vi "LabVIEW-CommEx_Bus_Interface_PWM_SPI_v1.1a_Scaled_6Apr2023.vi"() -> ()   [LabVIEW 2018]
uses:
  <vilib>/Instr/_visa.llb/VISA Set IO Buffer Mask.ctl
  <vilib>/Utility/error.llb/DialogType.ctl
  <vilib>/Instr/_visa.llb/VISA Configure Serial Port (Serial Instr).vi
panel:
  out "V_DC_In":dbl format="%.2f"
  out "V_Boost":dbl format="%.2f"
  out "V_Buck":dbl format="%.2f"
  out "V_Pot":dbl format="%.2f"
  in  "LED4_Intensity":dbl(slide)=100.0 scale=0.0..100.0
  in  "LED3_Intensity":dbl(slide)=50.0 scale=0.0..100.0
  in  "LED2_Intensity":dbl(slide)=25.0 scale=0.0..100.0
  in  "LED_BlinkPRD":dbl(slide)=75.0 scale=0.0..100.0
  in  "LED1_Intensity":dbl(slide)=12.5 scale=0.0..100.0
  in  "PWM_En":bool=TRUE
  out "error out 2":errorcluster={"status"=FALSE, "code"=1073676294, "source"="VISA Read in LabVIEW-Int_FPGA_CommExample_2Jun2019_v1.1a_2Jun2019.vi"}
  out "Reg_Array":u16[](array[numeric])=[1, 49151, 24576, 8192, 16384, 32768, 65535, 0, 0, 0, 0, 0, 0, 0, 0, 0, 0, 0, 0, 0, 0, 0, 0, 0, 0, 0, 0, 0, 0, 0, 0, 0, 0, 0, 0, 0, 0, 0, 0, 0, 0, 0, 0, 0, 0, 0, 0, 0, 0, 0, 0, 0, 0, 0, 0, 0, 0, 0, 0, 0, 0, 0, 0, 0] format="%x"
  out "Read_Packet":string
  out "CkSum":bool=TRUE
  out "Recieved Packet":string
  in  "flow control":u16(ring) items=["None"=0, "XON/XOFF"=1, "RTS/CTS"=2, "DTR/DSR"=4]
  in  "Input Buffer Size":u32=16484
  in  "stop 2":bool
  in  "timeout (ms)":u32=100000
  in  "stop bits":u16(ring)=10 items=["1.0"=10, "1.5"=15, "2.0"=20]
  in  "parity":u16(ring) items=["None", "Odd", "Even", "Mark", "Space"]
  in  "data bits":u16=8 min=5 max=8 step=1
  in  "VISA resource name":refnum<visa-resource-name>="COM4"
  in  "baud rate":u32=9600
  out "Cmd_Packet":string
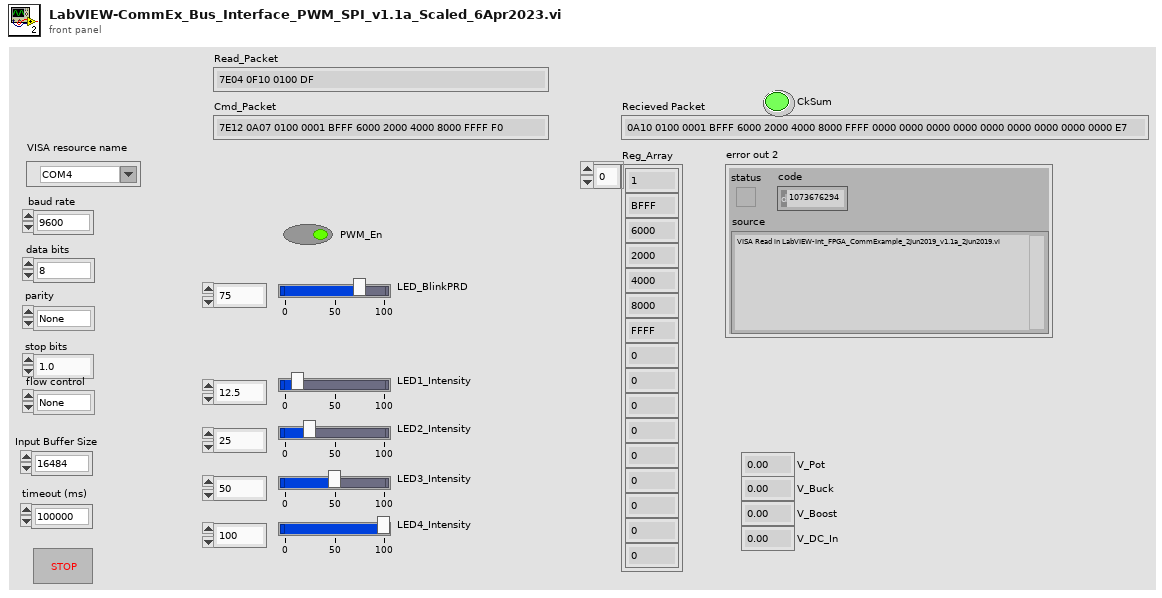
[diagram p1: front panel]
types:
  T1 = typedef "DialogType.ctl" = u16
  T2 = typedef "VISA Set IO Buffer Mask.ctl" = u16
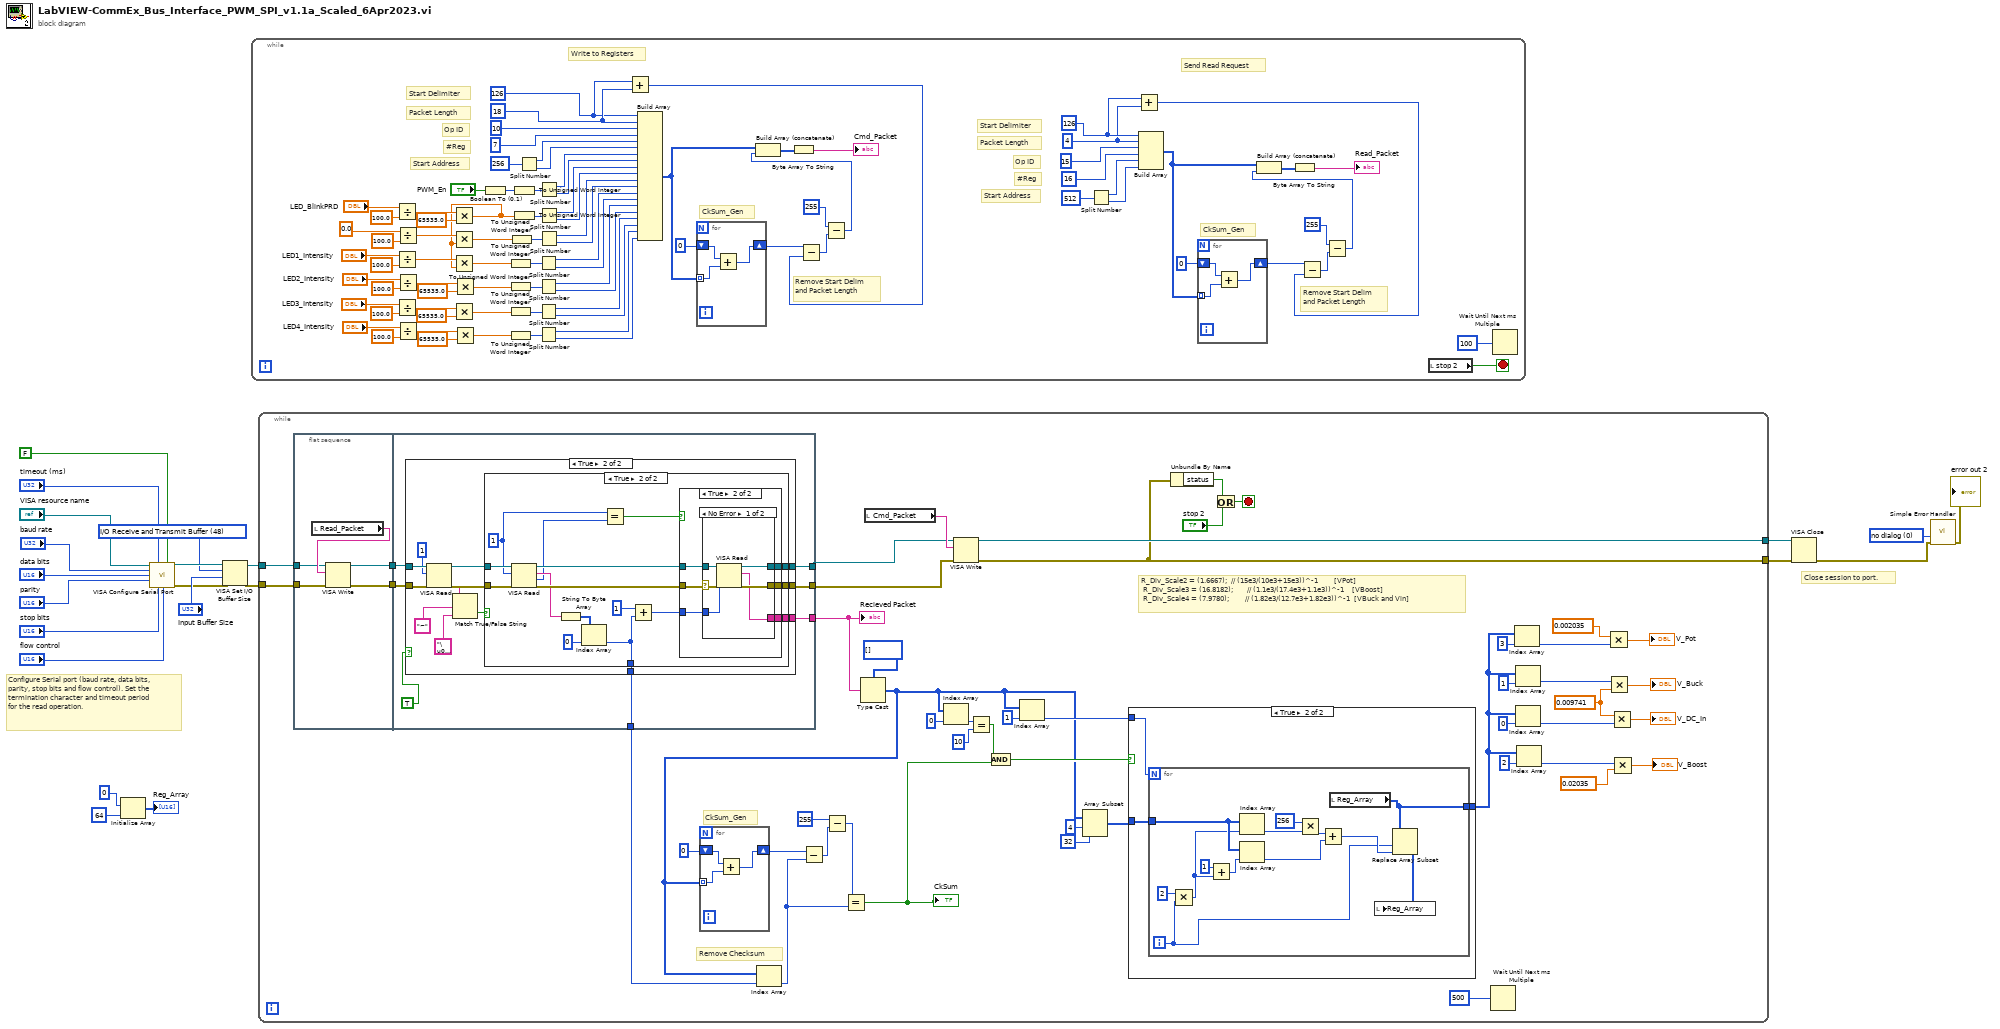
[diagram p0: block diagram]
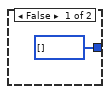
[diagram p2: hidden frame]
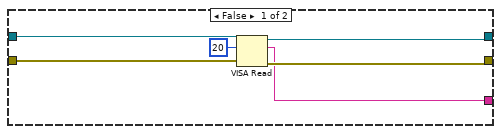
[diagram p3: hidden frame]
diagram:
  w2 = T1 0 items=["no dialog", "OK message", "continue or stop message", "OK message + warnings", "continue/stop + warnings"] ("type of dialog (OK msg:1)")
  w7 = T2 48 items=["I/O Receive Buffer"=16, "I/O Transmit Buffer"=32, "I/O Receive and Transmit Buffer"=48] ("Mask")
  # "Configure Serial port (baud rate, data bits, parity, stop bits and flow control). Set the termination character and timeout period for the read operation."
  # "Close session to port."
  n1 = Initialize Array(u16 0 ("element"), 64 ("dimension size")) -> (→"Reg_Array":u16[])
  n2 = call-poly "VISA Configure Serial Port"("VISA resource name"="VISA resource name", "timeout (10sec)"="timeout (ms)", "Enable Termination\nChar (T)"=FALSE, "baud rate (9600)"="baud rate", "data bits (8)"="data bits", "parity (0:none)"="parity", "stop bits (10: 1 bit)"="stop bits", "flow control (0:none)"="flow control") -> ("VISA resource name out"=w14:refnum<visa-resource-name>, "error out"=w13:errorcluster)  [unwired: 2 in, 4 out]
  n3 = VISA Set I/O Buffer Size(VISA resource name=w14, mask (16)=w7, size (4096)="Input Buffer Size", error in (no error)=w13) -> (VISA resource name out=w10:refnum<visa-resource-name>, error out=w11:errorcluster)
  n4 = while {
    stop <- w97 stop-if-true
    w26 = u8 4
    w27 = u8 126
    w80 = u8 18
    w79 = u8 126
    # "Write to Registers"
    # "Send Read Request"
    # "#Reg"
    # "Start Address"
    # "Start Delimiter"
    # "Packet Length"
    # "Op ID"
    # "Remove Start Delim\nand Packet Length"
    # "CkSum_Gen"
    # "Remove Start Delim\nand Packet Length"
    # "CkSum_Gen"
    # "#Reg"
    # "Start Address"
    # "Start Delimiter"
    # "Packet Length"
    # "Op ID"
    n5 = Divide(x="LED_BlinkPRD", y=100.0) -> (x/y=w60:dbl)
    n6 = Divide(x="LED1_Intensity", y=100.0) -> (x/y=w54:dbl)
    n7 = Divide(x="LED3_Intensity", y=100.0) -> (x/y=w43:dbl)
    n8 = Divide(x=0.0, y=100.0) -> (x/y=w57:dbl)
    n9 = Divide(x="LED2_Intensity", y=100.0) -> (x/y=w50:dbl)
    n10 = Divide(x="LED4_Intensity", y=100.0) -> (x/y=w38:dbl)
    n11 = Multiply(x=w60, y=65535.0 ("x")) -> (x*y=w23:dbl)
    n12 = Multiply(x=w57, y=w23) -> (x*y=w56:dbl)
    n13 = Multiply(x=w54, y=w23) -> (x*y=w53:dbl)
    n14 = Multiply(x=w43, y=65535.0 ("x")) -> (x*y=w41:dbl)
    n15 = Multiply(x=w50, y=65535.0 ("x")) -> (x*y=w47:dbl)
    n16 = Multiply(x=w38, y=65535.0 ("x")) -> (x*y=w35:dbl)
    n17 = Boolean To (0,1)(Boolean="PWM_En") -> (0, 1=w76:i16)
    n18 = To Unsigned Word Integer(number=w53) -> (unsigned 16bit integer=w93:u16)
    n19 = To Unsigned Word Integer(number=w47) -> (unsigned 16bit integer=w92:u16)
    n20 = To Unsigned Word Integer(number=w41) -> (unsigned 16bit integer=w46:u16)
    n21 = To Unsigned Word Integer(number=w35) -> (unsigned 16bit integer=w45:u16)
    n22 = To Unsigned Word Integer(number=w56) -> (unsigned 16bit integer=w94:u16)
    n23 = To Unsigned Word Integer(number=w76) -> (unsigned 16bit integer=w81:u16)
    n24 = To Unsigned Word Integer(number=w23) -> (unsigned 16bit integer=w107:u16)
    n25 = Split Number(x=u16 256) -> (hi(x)=w74:u8, lo(x)=w73:u8)
    n26 = Split Number(x=w93) -> (hi(x)=w66:u8, lo(x)=w65:u8)
    n27 = Split Number(x=w92) -> (hi(x)=w64:u8, lo(x)=w63:u8)
    n28 = Split Number(x=w46) -> (hi(x)=w34:u8, lo(x)=w33:u8)
    n29 = Split Number(x=w45) -> (hi(x)=w32:u8, lo(x)=w31:u8)
    n30 = Split Number(x=w81) -> (hi(x)=w72:u8, lo(x)=w71:u8)
    n31 = Split Number(x=w107) -> (hi(x)=w70:u8, lo(x)=w69:u8)
    n32 = Split Number(x=w94) -> (hi(x)=w68:u8, lo(x)=w67:u8)
    n33 = Add(x=w79, y=w80) -> (x+y=w78:u8)
    n34 = Build Array(w79, w80, u8 10, u8 7, w74, w73, w72, w71, w70, w69, w68, w67, w66, w65, w64, w63, w34, w33, w32, w31) -> (w104:u8[])
    n35 = for {
      tunnel: w104 -> [w111] mode=indexing
      shift-right: [w113] -> w96
      shift-left: u8 0 -> [w112]
      n36 = Add(x=w112, y=w111) -> (x+y=w113:u8)
    }
    n37 = Subtract(x=w96, y=w78) -> (x-y=w95:u8)
    n38 = Subtract(x=u8 255, y=w95) -> (x-y=w98:u8)
    n39 = Build Array (concatenate)(w104, w98) -> (w103:u8[])
    n40 = Byte Array To String(unsigned byte array=w103) -> (string=→"Cmd_Packet":string)
    n41 = Split Number(x=u16 512) -> (hi(x)=w29:u8, lo(x)=w28:u8)
    n42 = Add(x=w27, y=w26) -> (x+y=w25:u8)
    n43 = Build Array(w27, w26, u8 15, u8 16, w29, w28) -> (w90:u8[])
    n44 = for {
      tunnel: w90 -> [w108] mode=indexing
      shift-right: [w110] -> w85
      shift-left: u8 0 -> [w109]
      n45 = Add(x=w109, y=w108) -> (x+y=w110:u8)
    }
    n46 = Subtract(x=w85, y=w25) -> (x-y=w84:u8)
    n47 = Subtract(x=u8 255, y=w84) -> (x-y=w86:u8)
    n48 = Build Array (concatenate)(w90, w86) -> (w89:u8[])
    n49 = Byte Array To String(unsigned byte array=w89) -> (string=→"Read_Packet":string)
    n50 = local read "stop 2"() -> (w97:bool)
    n51 = Wait Until Next ms Multiple(millisecond multiple=u8 100) -> ()  [unwired: 1 out]
  }
  n52 = while {
    tunnel: w11 -> [w147]
    tunnel: w10 -> [w148]
    tunnel: [w152] -> w8
    tunnel: [w135] -> w9
    stop <- w162 stop-if-true
    w121 = 0.009741
    # "R_Div_Scale2 = (1.6667);\t\t// (15e3/(10e3+15e3))^-1        [VPot]\n\tR_Div_Scale3 = (16.8182);       // (1.1e3/(17.4e3+1.1e3))^-1    [VBoost]\n\tR_Div_Scale4 = (7.9780);        // (1.82e3/(12.7e3+1.82e3))^-1  [VBuck and Vin]"
    # "Remove Checksum"
    # "CkSum_Gen"
    n53 = flat-sequence {
      tunnel: [w184] -> w150
      tunnel: [w183] -> w149
      tunnel: w148 -> [w182]
      tunnel: w147 -> [w181]
      tunnel: [w192] -> w151
      tunnel: w150 -> [w191]
      tunnel: w149 -> [w190]
      tunnel: [w189] -> w146
      tunnel: [w188] -> w145
      tunnel: [w186] -> w138
      frame #0 {
        n54 = local read "Read_Packet"() -> (w185:string)
        n55 = VISA Write(VISA resource name=w182, write buffer=w185, error in (no error)=w181) -> (VISA resource name out=w184:refnum<visa-resource-name>, error out=w183:errorcluster)  [unwired: 1 out]
      }
      frame #1 {
        n56 = case shown="True" TRUE {
          tunnel: w190 -> [w197 w208]
          tunnel: w191 -> [w198 w206]
          tunnel: [w195 w211] -> w188
          tunnel: [w196 w210] -> w189
          tunnel: [w193 w209] -> w192
          tunnel: [_ w199] -> w186
          frame False {
            n57 = VISA Read(VISA resource name=w198, byte count=u32 20, error in (no error)=w197) -> (VISA resource name out=w196:refnum<visa-resource-name>, read buffer=w193:string, error out=w195:errorcluster)  [unwired: 1 out]
          }
          frame True {
            n58 = VISA Read(VISA resource name=w206, byte count=u32 1 ("millisecond multiple"), error in (no error)=w208) -> (VISA resource name out=w205:refnum<visa-resource-name>, read buffer=w203:string, error out=w207:errorcluster)  [unwired: 1 out]
            n59 = Match True/False String(2:"\u0000", 3:"~", 4:w203) -> (0:w201:bool)  [unwired: 1 out]
            n60 = case shown="True" w201 {
              tunnel: [w212 w229] -> w211
              tunnel: [w213 w228] -> w210
              tunnel: [_ w227] -> w209
              tunnel: w207 -> [w212 w226]
              tunnel: w205 -> [w213 w225]
              tunnel: [_ w214] -> w199
              frame False {
              }
              frame True {
                w218 = u32 1 ("byte count")
                n61 = VISA Read(VISA resource name=w225, byte count=w218, error in (no error)=w226) -> (VISA resource name out=w224:refnum<visa-resource-name>, read buffer=w221:string, return count=w217:u32, error out=w223:errorcluster)
                n62 = String To Byte Array(string=w221) -> (unsigned byte array=w220:u8[])
                n63 = Index Array(array=w220, index=u32 0 ("millisecond multiple")) -> (element=w214:u8)
                n64 = Equal?(x=w218, y=w217) -> (x = y?=w216:bool)
                n65 = Add(x=u32 1 ("millisecond multiple"), y=w214) -> (x+y=w215:u32)
                n66 = case shown="True" w216 {
                  tunnel: [w230 w237] -> w229
                  tunnel: [w231 w236] -> w228
                  tunnel: w223 -> [w230 w235]
                  tunnel: w224 -> [w231 w234]
                  tunnel: [_ w233] -> w227
                  tunnel: w215 -> [_ w232]
                  frame False {
                  }
                  frame True {
                    n67 = case "Read bytes from port." shown="No Error" w235 {
                      selector: w235 -> [w240 w244]
                      tunnel: [w242 w244] -> w237
                      tunnel: [w243 w245] -> w236
                      tunnel: w234 -> [w241 w245]
                      tunnel: [w238 _] -> w233
                      tunnel: w232 -> [w239 _]
                      frame No Error {
                        n68 = VISA Read(VISA resource name=w241, byte count=w239, error in (no error)=w240) -> (VISA resource name out=w243:refnum<visa-resource-name>, read buffer=w238:string, error out=w242:errorcluster)  [unwired: 1 out]
                      }
                      frame Error {
                        # "Error occurred \nreading Bytes at \nSerial Port"
                      }
                    }
                  }
                }
              }
            }
          }
        }
      }
    }
    n69 = Type Cast(type=u8[] [], x=w151) -> (*(type *) &x=w133:u8[])
    n70 = for {
      tunnel: w133 -> [w246] mode=indexing
      shift-right: [w248] -> w156
      shift-left: u8 0 -> [w247]
      n71 = Add(x=w247, y=w246) -> (x+y=w248:u8)
    }
    n72 = Index Array(array=w133, index=w138) -> (element=w153:u8)
    n73 = Subtract(x=w156, y=w153) -> (x-y=w155:u8)
    n74 = Subtract(x=u8 255, y=w155) -> (x-y=w154:u8)
    n75 = Equal?(x=w154, y=w153) -> (x = y?=w136:bool)
    "CkSum" <- w136
    n76 = local read "Cmd_Packet"() -> (w159:string)
    n77 = Index Array(array=w133, index=0) -> (element=w143:u8)
    n78 = VISA Write(VISA resource name=w146, write buffer=w159, error in (no error)=w145) -> (VISA resource name out=w152:refnum<visa-resource-name>, error out=w135:errorcluster)  [unwired: 1 out]
    n79 = Equal?(x=w143, y=u16 10) -> (x = y?=w141:bool)
    n80 = And(x=w141, y=w136) -> (x .and. y?=w140:bool)
    n81 = Index Array(array=w133, index=1) -> (element=w137:u8)
    n82 = Array Subset(array=w133, index=4, length=32) -> (w132:u8[])
    n83 = case shown="True" w140 {
      tunnel: w137 -> [_ w166]
      tunnel: w132 -> [_ w167]
      tunnel: [u16[] [] ("Reg_Array") w165] -> w117
      frame False {
      }
      frame True {
        n84 = for {
          N: w166 -> [_]
          tunnel: w167 -> [w176]
          tunnel: [w168] -> w165
          i -> [w172]
          n85 = Multiply(x=2, y=w172) -> (x*y=w171:i32)
          n86 = Add(x=1, y=w171) -> (x+y=w169:i32)
          n87 = Index Array(array=w176, index=w171) -> (element=w178:u8)
          n88 = Index Array(array=w176, index=w169) -> (element=w177:u8)
          n89 = Multiply(x=u32 256 ("millisecond multiple"), y=w178) -> (x*y=w180:u32)
          n90 = Add(x=w180, y=w177) -> (x+y=w175:u32)
          n91 = local read "Reg_Array"() -> (w168:u16[])
          n92 = Replace Array Subset(array=w168, new element=w175, index=w172) -> (w174:u16[])
          n93 = local write "Reg_Array"(w174) -> ()
        }
      }
    }
    n94 = Unbundle By Name(w135) -> ("status"=w163:bool)
    n95 = Or(x=w163, y="stop 2") -> (x .or. y?=w162:bool)
    n96 = Wait Until Next ms Multiple(millisecond multiple=u32 500) -> ()  [unwired: 1 out]
    n97 = Index Array(array=w117, index=3) -> (element=w123:u16)
    n98 = Index Array(array=w117, index=0) -> (element=w119:u16)
    n99 = Index Array(array=w117, index=1) -> (element=w120:u16)
    n100 = Index Array(array=w117, index=2) -> (element=w118:u16)
    n101 = Multiply(x=0.002035, y=w123) -> (x*y=→"V_Pot":dbl)
    n102 = Multiply(x=w120, y=w121) -> (x*y=→"V_Buck":dbl)
    n103 = Multiply(x=w121, y=w119) -> (x*y=→"V_DC_In":dbl)
    n104 = Multiply(x=w118, y=0.02035) -> (x*y=→"V_Boost":dbl)
    "Recieved Packet" <- w151
  }
  n105 = VISA Close(VISA resource name=w8, error in (no error)=w9) -> (error out=w1:errorcluster)
  n106 = call <vilib>:"Simple Error Handler.vi"("type of dialog (OK msg:1)"=w2, "error in (no error)"=w1) -> ("error out"=→"error out 2":errorcluster)  [unwired: 7 out]
